vi "3boolsToString.vi"(1 "input_bool_low":bool=TRUE, 2 "input_bool_mid":bool=TRUE, 3 "input_bool_high":bool=TRUE) -> (0 "show_str_011string":string)   [LabVIEW 2011]
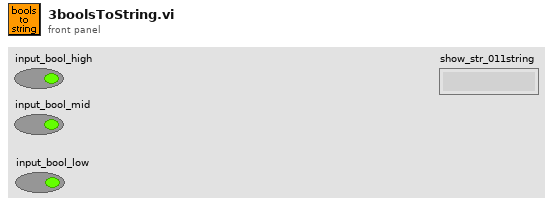
[diagram p1: front panel]
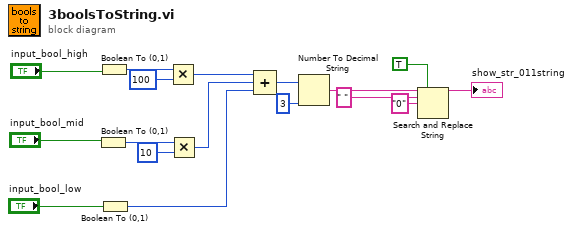
[diagram p0: block diagram]
diagram:
  n1 = Boolean To (0,1)(Boolean="input_bool_mid") -> (0, 1=w4:i16)
  n2 = Boolean To (0,1)(Boolean="input_bool_high") -> (0, 1=w15:i16)
  n3 = Boolean To (0,1)(Boolean="input_bool_low") -> (0, 1=w1:i16)
  n4 = Multiply(x=w15, y=i16 100) -> (x*y=w3:i16)
  n5 = Multiply(x=w4, y=i16 10) -> (x*y=w2:i16)
  n6 = Compound Arithmetic op=ADD(w3, w2, w1) -> (w13:i16)
  n7 = Number To Decimal String(number=w13, width (-)=i16 3 ("宽度(-)")) -> (decimal integer string=w11:string)
  n8 = Search and Replace String(replace all?=TRUE ("替换全部？(F)"), input string=w11, search string=" " ("搜索字符串"), replace string="0" ("替换字符串(\"\")")) -> (result string=→"show_str_011string":string)  [unwired: 4 in, 3 out]
